vi "SSFG_sharp_test.vi"() -> ()   [LabVIEW 2014]
uses:
  SSFG_States.ctl
  <vilib>/Utility/error.llb/DialogType.ctl
  <vilib>/DAQmx/write.llb/DAQmx Write (Analog Wfm 1Chan NSamp).vi
  <vilib>/DAQmx/read.llb/DAQmx Read (Analog Wfm 1Chan NSamp).vi
  <vilib>/DAQmx/create/channels.llb/DAQmx Create Channel (AO-Voltage-Basic).vi
  <vilib>/DAQmx/configure/timing.llb/DAQmx Timing (Sample Clock).vi
  <vilib>/DAQmx/create/channels.llb/DAQmx Create Channel (AI-Voltage-Basic).vi
  <vilib>/DAQmx/configure/trigger.llb/DAQmx Start Trigger (Digital Edge).vi
  <vilib>/DAQmx/miscellaneous.llb/DAQmx Fill In Error Info.vi
  <resource>/objmgr/daqmx.rc
  <vilib>/measure/NI_MABase.lvlib
panel:
  out "size(s)":i32
  in  "Physical Channel 2":tag="Dev1/ai0" caption="Physical Channel"
  in  "Sample Rate":dbl=10000.0 caption="Sample Rate (Hz)" format="%0.2f"
  out "Measurement":waveform(dbl)(graph)
  in  "stop 2":bool caption="stop"
  in  "Samples to Read":i32=1000
  out "cycle RMS":dbl format="%.2g"
  out "Numeric":i32
  out "Iterations":i32
  in  "Attenuation":dbl
  in  "Number of Samples/Cycle":dbl
  out "Generation":waveform(dbl)(graph)
  in  "stop":bool
  in  "Power Signal Parameters":T1={"Waveform Type"=0, "Amplitude"=1.0, "Frequency"=17.0} {"Frequency" format="%0.2p"; "Waveform Type" items=["Sine Wave", "Triangle Wave", "Square Wave", "Sawtooth Wave"]}
  out "Flicker":bool
  out "Swell":bool
  out "Sag":bool
  in  "Stop":bool
  in  "Update Rate":dbl=1000.0 format="%0.2f"
  in  "Generation":tag
  in  "Flicker":T2
  in  "Swell":cluster{"Swell_Time (sec)":dbl, "Swell":bool}
  in  "Sag":cluster{"Sag_Time (sec)":dbl, "Sag":bool}
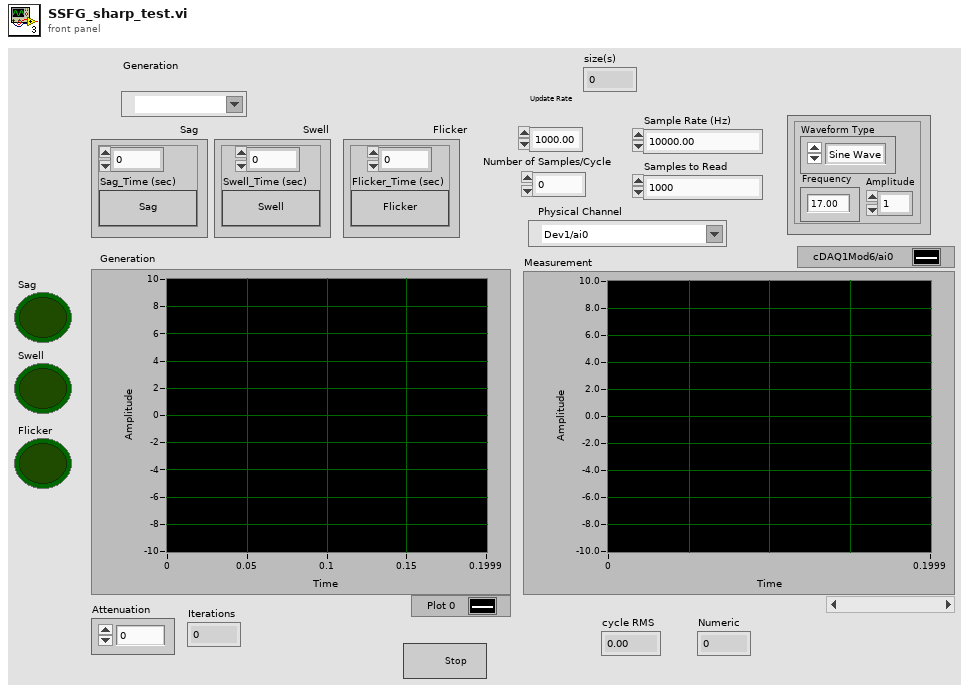
[diagram p1: front panel]
types:
  T1 = cluster{"Waveform Type":u16, "Amplitude":dbl, "Frequency":dbl}
  T2 = cluster{"Flicker_Time (sec)":dbl, "Flicker":bool}
  T3 = typedef "DialogType.ctl" = u16
  T4 = typedef "SSFG_States.ctl" = cluster{"State":string, "Disturbance_Time (sec)":dbl}
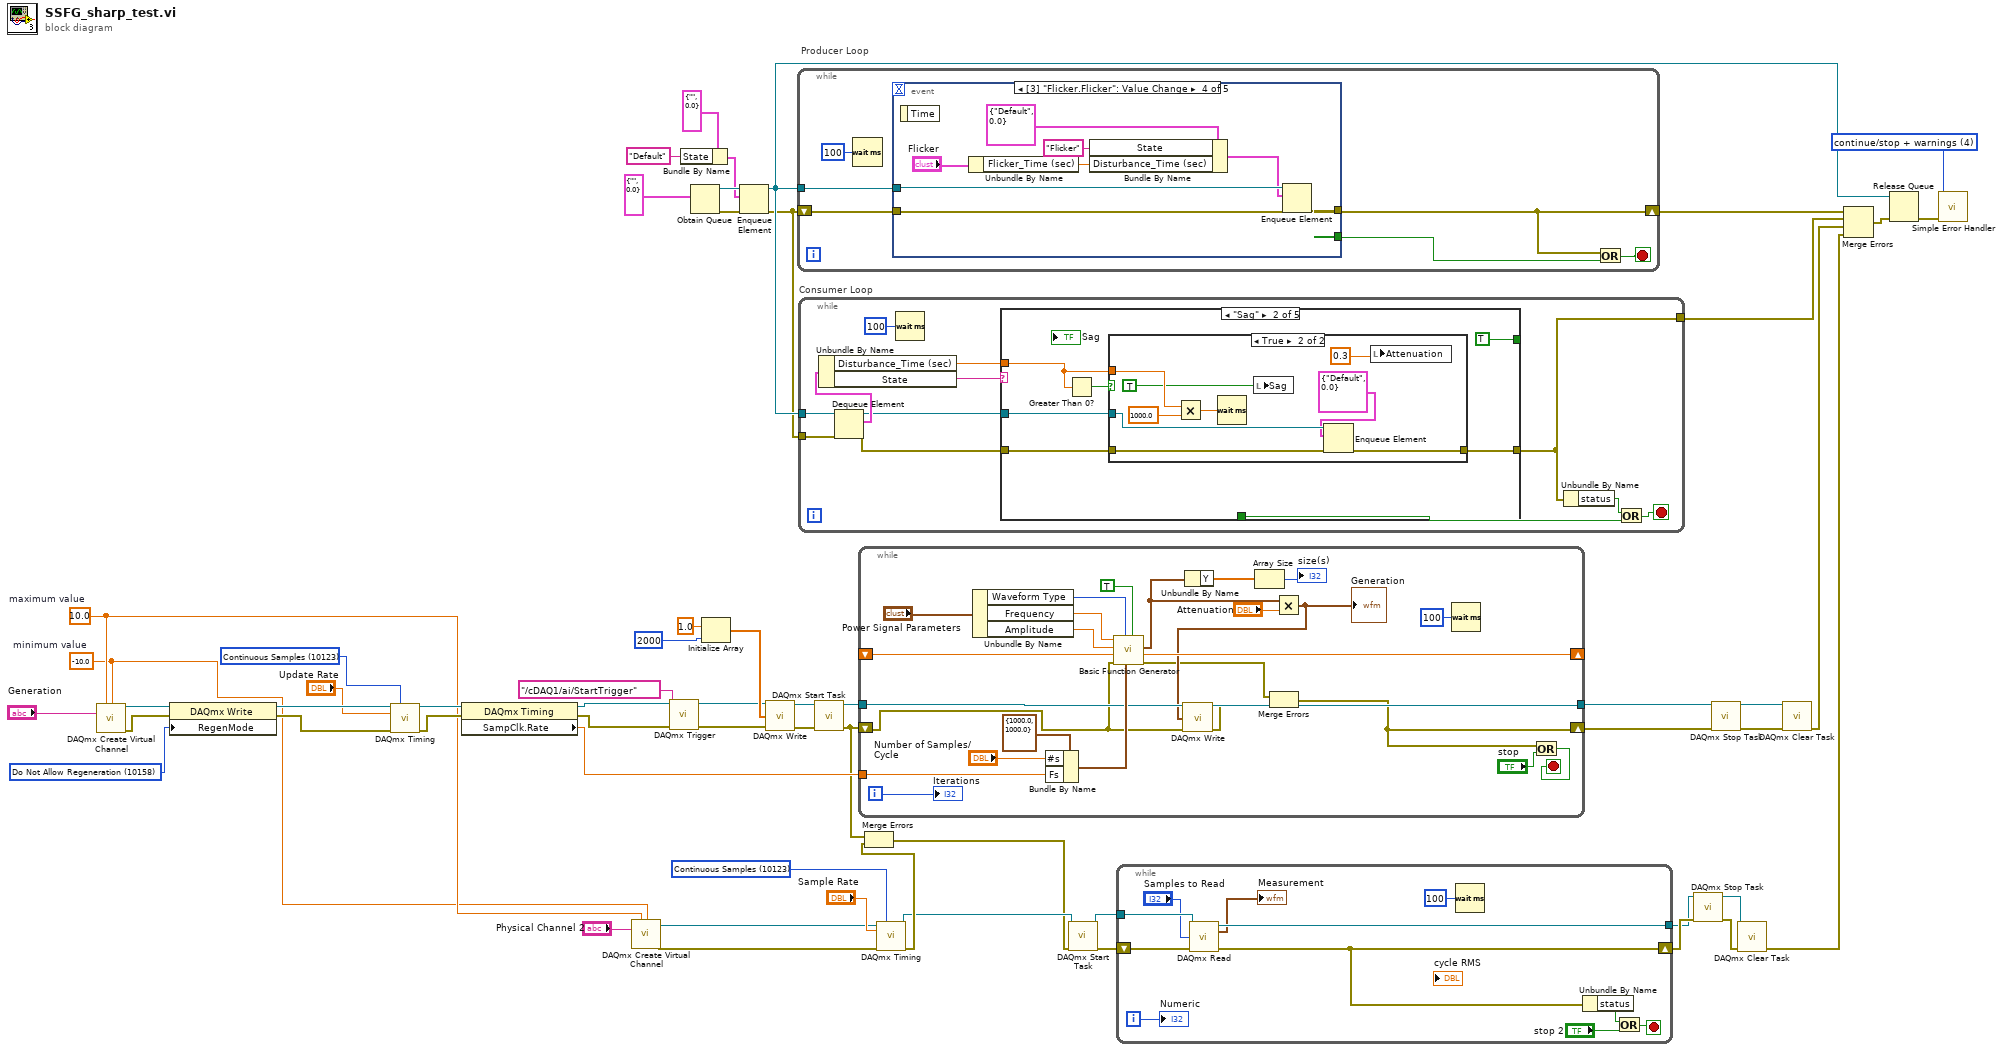
[diagram p0: block diagram]
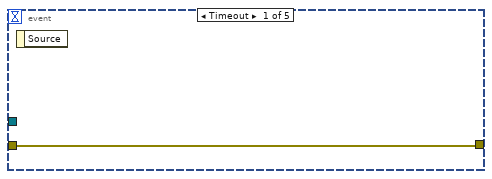
[diagram p2: hidden frame]
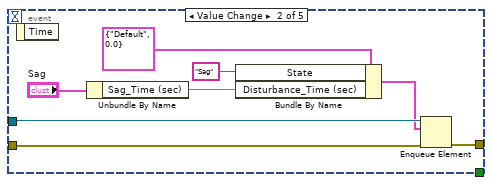
[diagram p3: hidden frame]
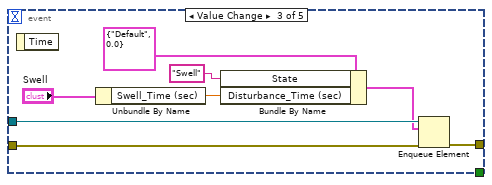
[diagram p4: hidden frame]
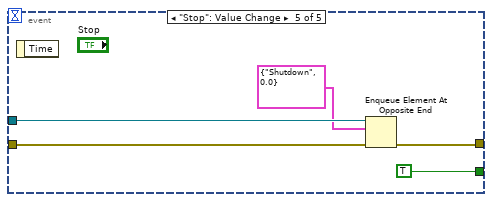
[diagram p5: hidden frame]
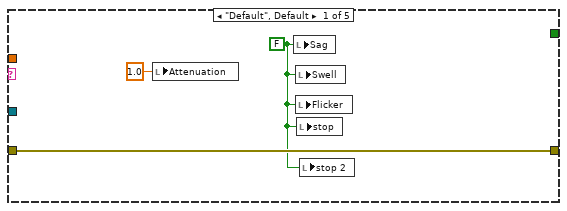
[diagram p6: hidden frame]
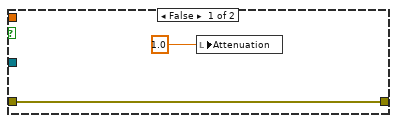
[diagram p7: hidden frame]
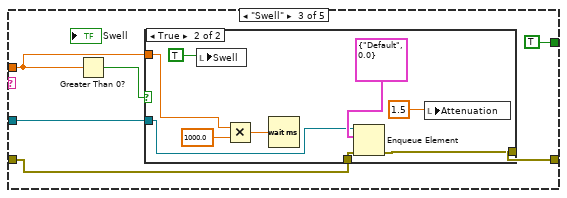
[diagram p8: hidden frame]
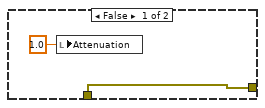
[diagram p9: hidden frame]
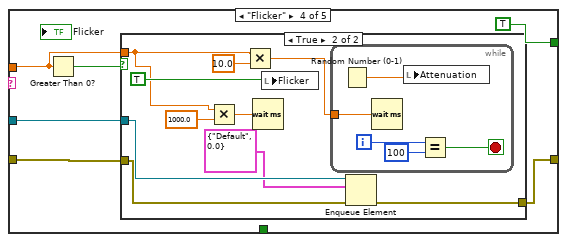
[diagram p10: hidden frame]
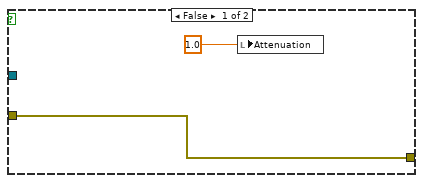
[diagram p11: hidden frame]
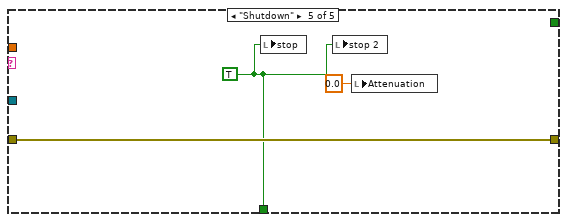
[diagram p12: hidden frame]
diagram:
  w5 = T3 4 items=["no dialog", "OK message", "continue or stop message", "OK message + warnings", "continue/stop + warnings"] ("type of dialog (OK msg:1)")
  w41 = 10123 items=["Finite Samples"=10178, "Continuous Samples"=10123] ("sample mode")
  w36 = 10.0  # maximum value
  w35 = -10.0  # minimum value
  w52 = 10123 items=["Finite Samples"=10178, "Continuous Samples"=10123, "Hardware Timed Single Point"=12522] ("sample mode")
  w53 = 10158 items=["Allow Regeneration"=10097, "Do Not Allow Regeneration"=10158] ("RegenMode")
  n1 = call-poly <vilib>:"DAQmx Create Virtual Channel.vi"("maximum value"=w36, "minimum value"=w35, "physical channels"="Generation") -> ("task out"=w57:refnum<k21>, "error out"=w55:errorcluster)  [unwired: 11 in]
  n2 = property class="DAQmx Write"(reference=w57, error in=w55, "RegenMode"=w53) -> (reference out=w56:refnum<k21>, error out=w54:errorcluster)
  n3 = call-poly <vilib>:"DAQmx Timing.vi"("task/channels in"=w56, "sample mode"=w52, "rate"="Update Rate", "error in"=w54) -> ("task out"=w46:refnum<k21>, "error out"=w45:errorcluster)  [unwired: 10 in]
  n4 = property class="DAQmx Timing"(reference=w46, error in=w45) -> (reference out=w31:refnum<k21>, error out=w29:errorcluster, "SampClk.Rate"=w49:dbl)
  n5 = call-poly <vilib>:"DAQmx Create Virtual Channel.vi"("maximum value"=w36, "minimum value"=w35, "physical channels"="Physical Channel 2") -> ("task out"=w38:refnum<k21>, "error out"=w37:errorcluster)  [unwired: 11 in]
  n6 = call-poly <vilib>:"DAQmx Trigger.vi"("task/channels in"=w31, "source"=tag "/cDAQ1/ai/StartTrigger", "error in"=w29) -> ("task out"=w30:refnum<k21>, "error out"=w28:errorcluster)  [unwired: 11 in]
  n7 = Bundle By Name(cluster=T4 {"State"="", "Disturbance_Time (sec)"=0.0}, "State"="Default") -> (w10:T4)
  n8 = Obtain Queue(element data type=T4 {"State"="", "Disturbance_Time (sec)"=0.0}) -> (queue out=w14:refnum<queue>, error out=w13:errorcluster)  [unwired: 4 in, 1 out]
  n9 = Initialize Array(1.0 ("element"), 2000 ("dimension size")) -> (w32:dbl[])
  n10 = Enqueue Element(queue=w14, element=w10, error in (no error)=w13) -> (queue out=w8:refnum<queue>, error out=w7:errorcluster)  [unwired: 1 in, 1 out]
  n11 = call-poly <vilib>:"DAQmx Write.vi"("task/channels in"=w30, "data"=w32, "error in"=w28) -> ("task out"=w26:refnum<k21>, "error out"=w23:errorcluster)  [unwired: 10 in, 1 out]
  n12 = while "Producer Loop" {
    tunnel: w8 -> [w63]
    shift-right: [w61] -> w16
    shift-left: w7 -> [w62]
    stop <- w64 stop-if-true
    n13 = Wait (ms)(milliseconds to wait=u32 100) -> ()  [unwired: 1 out]
    n14 = event shown="[3] \"Flicker.Flicker\": Value Change" {
      selector: _ -> [_ _ _ _ _]
      dyn-events: _ -> [_ _ _ _ _]
      timeout: _ -> [_ _ _ _ _]
      tunnel: w63 -> [_ w73 w81 w89 w94]
      tunnel: w62 -> [w65 w72 w80 w88 w93]
      tunnel: [w65 w71 w79 w87 w92] -> w61
      tunnel: [_ _ _ _ TRUE] -> w60
      event Timeout {
        n15 = event-data() -> ()  [unwired: 1 in, 1 out]
      }
      event "Sag.Sag": Value Change {
        n16 = event-data() -> ()  [unwired: 1 in, 1 out]
        n17 = Unbundle By Name("Sag") -> ("Sag_Time (sec)"=w68:dbl)
        n18 = Bundle By Name(cluster=T4 {"State"="Default", "Disturbance_Time (sec)"=0.0}, "State"="Sag", "Disturbance_Time (sec)"=w68) -> (w67:T4)
        n19 = Enqueue Element(queue=w73, element=w67, error in (no error)=w72) -> (error out=w71:errorcluster)  [unwired: 1 in, 2 out]
      }
      event "Swell.Swell": Value Change {
        n20 = event-data() -> ()  [unwired: 1 in, 1 out]
        n21 = Unbundle By Name("Swell") -> ("Swell_Time (sec)"=w77:dbl)
        n22 = Bundle By Name(cluster=T4 {"State"="Default", "Disturbance_Time (sec)"=0.0}, "State"="Swell", "Disturbance_Time (sec)"=w77) -> (w75:T4)
        n23 = Enqueue Element(queue=w81, element=w75, error in (no error)=w80) -> (error out=w79:errorcluster)  [unwired: 1 in, 2 out]
      }
      event "Flicker.Flicker": Value Change {
        n24 = event-data() -> ()  [unwired: 1 in, 1 out]
        n25 = Unbundle By Name("Flicker") -> ("Flicker_Time (sec)"=w84:dbl)
        n26 = Bundle By Name(cluster=T4 {"State"="Default", "Disturbance_Time (sec)"=0.0}, "State"="Flicker", "Disturbance_Time (sec)"=w84) -> (w83:T4)
        n27 = Enqueue Element(queue=w89, element=w83, error in (no error)=w88) -> (error out=w87:errorcluster)  [unwired: 1 in, 2 out]
      }
      event "Stop": Value Change {
        n28 = event-data() -> ()  [unwired: 1 in, 1 out]
        n29 = Enqueue Element At Opposite End(queue=w94, element=T4 {"State"="Shutdown", "Disturbance_Time (sec)"=0.0}, error in (no error)=w93) -> (error out=w92:errorcluster)  [unwired: 1 in, 2 out]
      }
    }
    n30 = Or(x=w61, y=w60) -> (x .or. y?=w64:bool)
  }
  n31 = while "Consumer Loop" {
    tunnel: [w99] -> w6
    tunnel: w8 -> [w104]
    tunnel: w7 -> [w103]
    stop <- w106 stop-if-true
    n32 = Dequeue Element(queue=w104, error in (no error)=w103) -> (queue out=w98:refnum<queue>, element=w102:T4, error out=w97:errorcluster)  [unwired: 1 in, 1 out]
    n33 = Unbundle By Name(w102) -> ("Disturbance_Time (sec)"=w96:dbl, "State"=w101:string)
    n34 = Wait (ms)(milliseconds to wait=u32 100) -> ()  [unwired: 1 out]
    n35 = case shown="\"Sag\"" w101 {
      tunnel: [_ _ _ _ w167] -> w100
      tunnel: w97 -> [w109 w112 w130 w147 w168]
      tunnel: [w109 w113 w129 w146 w168] -> w99
      tunnel: w98 -> [_ w111 w128 w145 _]
      tunnel: w96 -> [_ w114 w131 w148 _]
      tunnel: [_ TRUE TRUE TRUE _] -> _
      frame "Default", Default {
        w107 = FALSE ("Sag")
        n36 = local write "Attenuation"(1.0 ("Attenuation")) -> ()
        n37 = local write "Sag"(w107) -> ()
        n38 = local write "Swell"(w107) -> ()
        n39 = local write "Flicker"(w107) -> ()
        n40 = local write "stop"(w107) -> ()
        n41 = local write "stop 2"(w107) -> ()
      }
      frame "Sag" {
        n42 = Greater Than 0?(x=w114) -> (x > 0?=w115:bool)
        n43 = case shown="True" w115 {
          tunnel: w114 -> [_ w120]
          tunnel: [w116 w125] -> w113
          tunnel: w112 -> [w116 w124]
          tunnel: w111 -> [_ w123]
          frame False {
            n44 = local write "Attenuation"(1.0 ("y")) -> ()
          }
          frame True {
            n45 = Multiply(x=w120, y=1000.0) -> (x*y=w121:dbl)
            n46 = Wait (ms)(milliseconds to wait=w121) -> ()  [unwired: 1 out]
            n47 = local write "Sag"(TRUE ("Auto Reset")) -> ()
            n48 = Enqueue Element(queue=w123, element=T4 {"State"="Default", "Disturbance_Time (sec)"=0.0}, error in (no error)=w124) -> (error out=w125:errorcluster)  [unwired: 1 in, 2 out]
            n49 = local write "Attenuation"(0.3 ("y")) -> ()
          }
        }
      }
      frame "Swell" {
        n50 = Greater Than 0?(x=w131) -> (x > 0?=w132:bool)
        n51 = case shown="True" w132 {
          tunnel: w131 -> [_ w138]
          tunnel: w130 -> [w133 w142]
          tunnel: [w133 w141] -> w129
          tunnel: w128 -> [_ w136]
          frame False {
            n52 = local write "Attenuation"(1.0 ("y")) -> ()
          }
          frame True {
            n53 = local write "Swell"(TRUE ("Auto Reset")) -> ()
            n54 = Multiply(x=w138, y=1000.0) -> (x*y=w140:dbl)
            n55 = Wait (ms)(milliseconds to wait=w140) -> ()  [unwired: 1 out]
            n56 = Enqueue Element(queue=w136, element=T4 {"State"="Default", "Disturbance_Time (sec)"=0.0}, error in (no error)=w142) -> (error out=w141:errorcluster)  [unwired: 1 in, 2 out]
            n57 = local write "Attenuation"(1.5 ("y")) -> ()
          }
        }
      }
      frame "Flicker" {
        n58 = Greater Than 0?(x=w148) -> (x > 0?=w149:bool)
        n59 = case shown="True" w149 {
          tunnel: w148 -> [_ w153]
          tunnel: w147 -> [w150 w161]
          tunnel: [w150 w160] -> w146
          tunnel: w145 -> [_ w159]
          frame False {
            n60 = local write "Attenuation"(1.0 ("y")) -> ()
          }
          frame True {
            n61 = Multiply(x=w153, y=1000.0) -> (x*y=w157:dbl)
            n62 = Multiply(x=w153, y=10.0) -> (x*y=w152:dbl)
            n63 = Wait (ms)(milliseconds to wait=w157) -> ()  [unwired: 1 out]
            n64 = local write "Flicker"(TRUE ("Auto Reset")) -> ()
            n65 = while {
              tunnel: w152 -> [w166]
              i -> [w164]
              stop <- w163 stop-if-true
              n66 = Random Number (0-1)() -> (number: 0 to 1=w165:dbl)
              n67 = Wait (ms)(milliseconds to wait=w166) -> ()  [unwired: 1 out]
              n68 = local write "Attenuation"(w165) -> ()
              n69 = Equal?(x=w164, y=100) -> (x = y?=w163:bool)
            }
            n70 = Enqueue Element(queue=w159, element=T4 {"State"="Default", "Disturbance_Time (sec)"=0.0}, error in (no error)=w161) -> (error out=w160:errorcluster)  [unwired: 1 in, 2 out]
          }
        }
      }
      frame "Shutdown" {
        w167 = TRUE
        n71 = local write "stop"(w167) -> ()
        n72 = local write "stop 2"(w167) -> ()
        n73 = local write "Attenuation"(0.0 ("Attenuation")) -> ()
      }
    }
    n74 = Unbundle By Name(w99) -> ("status"=w105:bool)
    n75 = Or(x=w105, y=w100) -> (x .or. y?=w106:bool)
  }
  n76 = call <vilib>:"DAQmx Start Task.vi"("task/channels in"=w26, "error in"=w23) -> ("task out"=w25:refnum<k21>, "error out"=w22:errorcluster)  [unwired: 12 in]
  n77 = while {
    tunnel: [w194] -> w50
    tunnel: w25 -> [w181]
    tunnel: w49 -> [w187]
    shift-right: [w185] -> _
    shift-left: _ -> [w184]
    shift-right: [w171] -> w20
    shift-left: w22 -> [w180]
    i -> [w182]
    stop <- w178 stop-if-true
    n78 = Unbundle By Name("Power Signal Parameters") -> ("Waveform Type"=w193:u16, "Frequency"=w192:dbl, "Amplitude"=w191:dbl)
    n79 = Bundle By Name(cluster=cluster{"Fs":dbl, "#s":dbl} {"Fs"=1000.0, "#s"=1000.0} ("sampling info"), "#s"="Number of Samples/Cycle", "Fs"=w187) -> (w188:cluster{"Fs":dbl, "#s":dbl})
    n80 = call <vilib>:"Basic Function Generator.vi"("reset signal"=TRUE, "sampling info"=w188, "signal type"=w193, "error in (no error)"=w180, "phase"=w184, "amplitude"=w191, "frequency"=w192) -> ("error out"=w172:errorcluster, "phase out"=w185:dbl, "signal out"=w176:waveform(dbl))  [unwired: 2 in]
    n81 = Unbundle By Name(w176) -> ("Y"=w175:dbl[])
    n82 = Array Size(array=w175) -> (size(s)=→"size(s)":i32)
    n83 = Multiply(x=w176, y="Attenuation") -> (x*y=w177:waveform(dbl))
    "Generation" <- w177
    n84 = call-poly <vilib>:"DAQmx Write.vi"("task/channels in"=w181, "data"=w177, "error in"=w180) -> ("task out"=w194:refnum<k21>, "error out"=w173:errorcluster)  [unwired: 10 in, 1 out]
    n85 = Merge Errors(w172, w173) -> (w171:errorcluster)
    n86 = Wait (ms)(milliseconds to wait=u32 100) -> ()  [unwired: 1 out]
    n87 = Or(x=w171, y="stop") -> (x .or. y?=w178:bool)
    "Iterations" <- w182
  }
  n88 = call-poly <vilib>:"DAQmx Timing.vi"("task/channels in"=w38, "sample mode"=w41, "rate"="Sample Rate", "error in"=w37) -> ("task out"=w43:refnum<k21>, "error out"=w44:errorcluster)  [unwired: 10 in]
  n89 = Merge Errors(w22, w44) -> (w21:errorcluster)
  n90 = call <vilib>:"DAQmx Start Task.vi"("task/channels in"=w43, "error in"=w21) -> ("task out"=w39:refnum<k21>, "error out"=w24:errorcluster)  [unwired: 12 in]
  n91 = while {
    tunnel: w39 -> [w205]
    tunnel: [w204] -> w3
    shift-right: [w201] -> w4
    shift-left: w24 -> [w206]
    i -> [w202]
    stop <- w198 stop-if-true
    n92 = call-poly <vilib>:"DAQmx Read.vi"("task/channels in"=w205, "number of samples per channel"="Samples to Read", "error in"=w206) -> ("task out"=w204:refnum<k21>, "data"=→"Measurement":waveform(dbl), "error out"=w201:errorcluster)  [unwired: 10 in]
    n93 = Wait (ms)(milliseconds to wait=u32 100) -> ()  [unwired: 1 out]
    n94 = Unbundle By Name(w201) -> ("status"=w199:bool)
    n95 = Or(x=w199, y="stop 2") -> (x .or. y?=w198:bool)
    "Numeric" <- w202
  }
  n96 = call <vilib>:"DAQmx Stop Task.vi"("task/channels in"=w3, "error in"=w4) -> ("task out"=w1:refnum<k21>, "error out"=w2:errorcluster)  [unwired: 12 in]
  n97 = call <vilib>:"DAQmx Stop Task.vi"("task/channels in"=w50, "error in"=w20) -> ("task out"=w48:refnum<k21>, "error out"=w47:errorcluster)  [unwired: 12 in]
  n98 = call <vilib>:"DAQmx Clear Task.vi"("task in"=w1, "error in"=w2) -> ("error out"=w19:errorcluster)  [unwired: 13 in]
  n99 = call <vilib>:"DAQmx Clear Task.vi"("task in"=w48, "error in"=w47) -> ("error out"=w18:errorcluster)  [unwired: 13 in]
  n100 = Merge Errors(w16, w6, w18, w19) -> (w15:errorcluster)
  n101 = Release Queue(queue=w8, error in (no error)=w15) -> (error out=w17:errorcluster)  [unwired: 1 in, 2 out]
  n102 = call <vilib>:"Simple Error Handler.vi"("type of dialog (OK msg:1)"=w5, "error in (no error)"=w17) -> ()  [unwired: 3 in, 5 out]
